vi "FTW-TestExecutive-Core_OnStartSequence.vi"(0 "FTW-TestExecutive-Core In":refnum<class "FTW-TestExecutive-Core.lvclass">, 11 "error in":errorcluster) -> (4 "FTW-TestExecutive-Core Out":refnum<class "FTW-TestExecutive-Core.lvclass">, 15 "error out":errorcluster)   [LabVIEW 2015, in "FTW-TestExecutive-Core.lvclass"]
uses:
  FTW-TestExecutive-Core.lvclass
  FTW-TestExecutive-Core.lvclass/FTW-TestExecutive-Core.ctl
  Instance/FTW-ActorInstance.lvclass
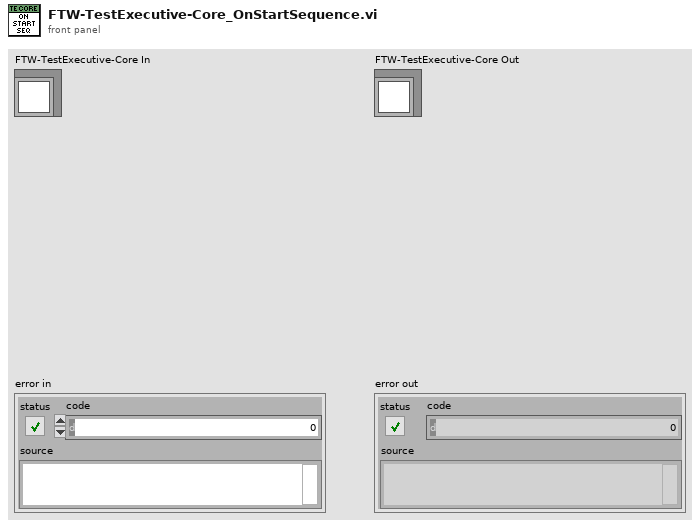
[diagram p1: front panel]
types:
  T1 = typedef "FTW-TestExecutive-Step.ctl" = cluster{"Name":string, "Type":string, "Config":string, "Elapsed Time":dbl, "Passed":bool, "State":T2, "Results":T3}
  T2 = typedef "FTW-TestExecutive-Step-State.ctl" = enum8{"None", "Failed", "Passed", "Timed out", "Aborted"}
  T3 = typedef "FTW-TestExecutive-Results.ctl" = cluster{"Start Time":timestamp, "Elapsed Time":dbl, "Passed":bool, "Additional Results":string}
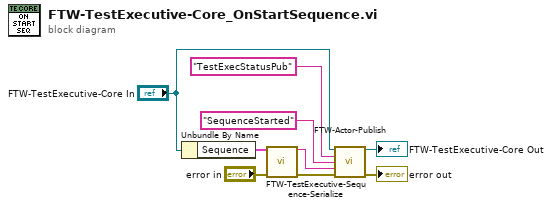
[diagram p0: block diagram]
diagram:
  n1 = Unbundle By Name("FTW-TestExecutive-Core In") -> ("Sequence"=w1:T1[])
  n2 = call "FTW-TestExecutive-Sequence-Serialize.vi"("Sequence"=w1, "error in"="error in") -> ("JSON"=w2:string, "error out"=w3:errorcluster)  [unwired: 12 in]
  n3 = call "FTW-Actor-Publish.vi"("FTW-ActorExtended In"="FTW-TestExecutive-Core In", "Publisher Name"="TestExecStatusPub", "Message Header"="SequenceStarted", "Message Body"=w2, "error in"=w3) -> ("FTW-ActorExtended Out"=→"FTW-TestExecutive-Core Out":refnum<class "FTW-TestExecutive-Core.lvclass">, "error out"=→"error out":errorcluster)  [unwired: 9 in]
